vi "PrepareBotsData.vi"(8 "error in (no error)":errorcluster, 11 "Game in":refnum<class "Game.lvclass">) -> (0 "error out":errorcluster, 1 "Bot2Data":T1, 2 "Bot1Data":T1, 3 "Game out":refnum<class "Game.lvclass">)   [LabVIEW 2015, in "TronviewGame.lvlib" / "Game.lvclass"]
uses:
  Game.lvclass
  TronVIEWBotAPI/BotData.ctl
  Game.lvclass/Game.ctl
  TronVIEWBotAPI/TronVIEWBotAPI.lvlib
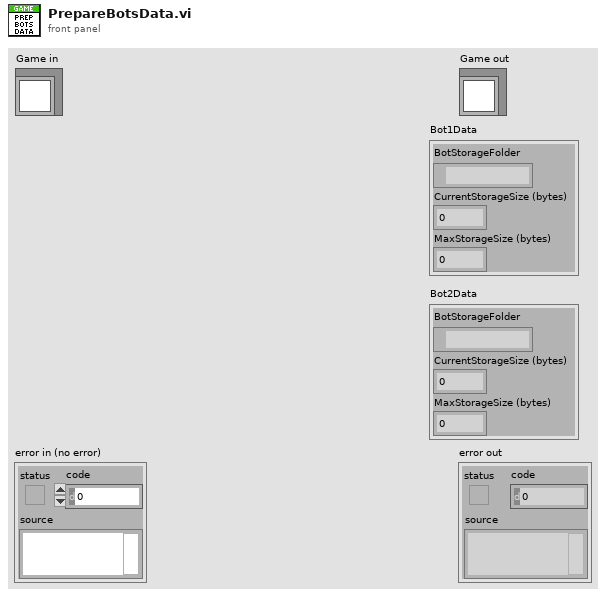
[diagram p1: front panel]
types:
  T1 = typedef "TronVIEWBotAPI.lvlib/BotData.ctl" = cluster{"BotStorageFolder":path, "CurrentStorageSize (bytes)":i64, "MaxStorageSize (bytes)":i64}
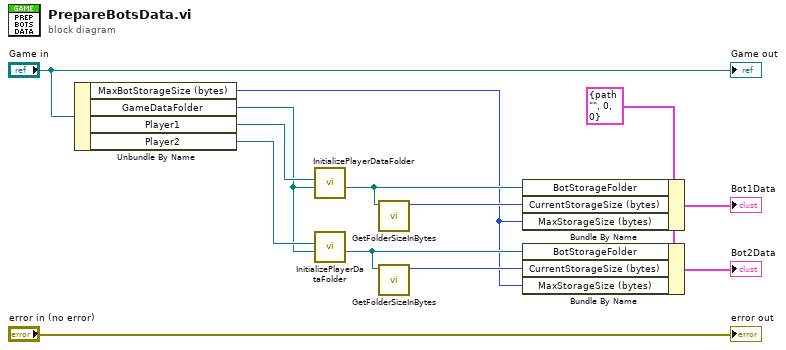
[diagram p0: block diagram]
diagram:
  w8 = T1 {"BotStorageFolder"=path "", "CurrentStorageSize (bytes)"=0, "MaxStorageSize (bytes)"=0} ("Bot1Data")
  n1 = Unbundle By Name("Game in") -> ("MaxBotStorageSize (bytes)"=w3:i64, "GameDataFolder"=w9:path, "Player1"=w11:refnum<class "Player.lvclass">, "Player2"=w10:refnum<class "Player.lvclass">)
  n2 = call "InitializePlayerDataFolder.vi"("BaseDataFolder"=w9, "Player in"=w11) -> ("PlayerDataPath"=w7:path)  [unwired: 7 in, 2 out]
  n3 = call "InitializePlayerDataFolder.vi"("BaseDataFolder"=w9, "Player in"=w10) -> ("PlayerDataPath"=w5:path)  [unwired: 7 in, 2 out]
  n4 = call "GetFolderSizeInBytes.vi"("Folder"=w7) -> ("FolderSize (bytes)"=w6:i64)  [unwired: 9 in, 1 out]
  n5 = call "GetFolderSizeInBytes.vi"("Folder"=w5) -> ("FolderSize (bytes)"=w4:i64)  [unwired: 9 in, 1 out]
  n6 = Bundle By Name(cluster=w8, "BotStorageFolder"=w7, "CurrentStorageSize (bytes)"=w6, "MaxStorageSize (bytes)"=w3) -> (→"Bot1Data":T1)
  n7 = Bundle By Name(cluster=w8, "BotStorageFolder"=w5, "CurrentStorageSize (bytes)"=w4, "MaxStorageSize (bytes)"=w3) -> (→"Bot2Data":T1)
  "error out" <- "error in (no error)"
  "Game out" <- "Game in"
